vi "Rectangle Set (SubVI).vi"(0 "x":dbl, 1 "x in":dbl, 2 "y":sgl, 3 "alpha":dbl format="%#_13g", 5 "y in":dbl=60.0 format="%#_13g") -> ()   [LabVIEW 2017]
uses:
  Projects/Auto control/Outputs.vi
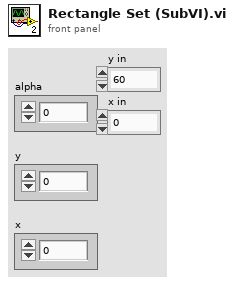
[diagram p1: front panel]
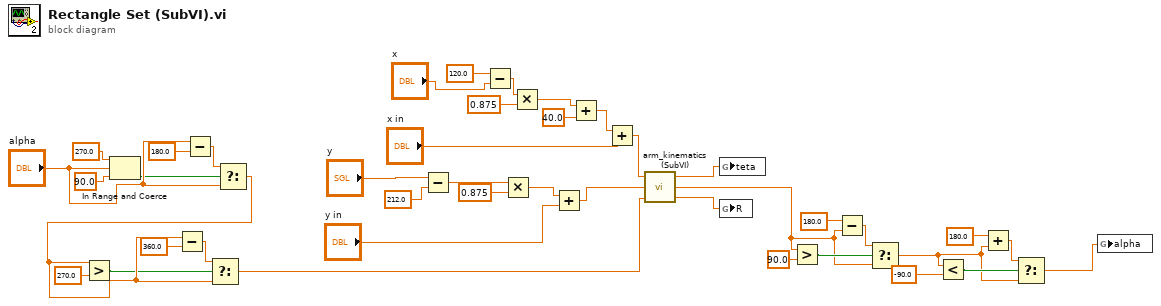
[diagram p0: block diagram]
diagram:
  n1 = In Range and Coerce(upper limit=270.0, x="alpha", lower limit=90.0) -> (In Range?=w28:bool)  [unwired: 1 out]
  n2 = Subtract(x="alpha", y=180.0) -> (x-y=w31:dbl)
  n3 = Select(t=w31, s=w28, f="alpha") -> (s? t:f=w37:dbl)
  n4 = Greater?(x=w37, y=270.0) -> (0:w36:bool)
  n5 = Subtract(x=w37, y=360.0) -> (x-y=w34:dbl)
  n6 = Select(t=w34, s=w36, f=w37) -> (s? t:f=w40:dbl)
  n7 = Subtract(x="y", y=sgl 212.0) -> (x-y=w24:sgl)
  n8 = Subtract(x=120.0, y="x") -> (x-y=w26:dbl)
  n9 = Multiply(x=w24, y=0.875) -> (x*y=w3:dbl)
  n10 = Multiply(x=w26, y=0.875) -> (x*y=w27:dbl)
  n11 = Add(x=w3, y="y in") -> (x+y=w2:dbl)
  n12 = Add(x=w27, y=40.0) -> (x+y=w6:dbl)
  n13 = Add(x=w6, y="x in") -> (x+y=w5:dbl)
  n14 = call "arm_kinematics (SubVI).vi"("alpha"=w40, "y"=w2, "x"=w5) -> ("R"=w18:dbl, "alpha"=w8:dbl, "teta"=w19:dbl)
  n15 = global write "Outputs.vi" "teta"(w19) -> ()
  n16 = global write "Outputs.vi" "R"(w18) -> ()
  n17 = Greater?(x=w8, y=90.0) -> (0:w16:bool)
  n18 = Subtract(x=180.0 ("y"), y=w8) -> (x-y=w15:dbl)
  n19 = Select(t=w15, s=w16, f=w8) -> (s? t:f=w9:dbl)
  n20 = Less?(x=w9, y=-90.0) -> (x < y?=w12:bool)
  n21 = Add(x=180.0 ("y"), y=w9) -> (x+y=w11:dbl)
  n22 = Select(t=w11, s=w12, f=w9) -> (s? t:f=w7:dbl)
  n23 = global write "Outputs.vi" "alpha"(w7) -> ()
